vi "Get Diagnostics.vi"(8 "error in (no error)":errorcluster, 11 "Red Pitaya Digitizer in":refnum<class "Red Pitaya Digitizer.lvclass">) -> (0 "error out":errorcluster, 2 "Diagnostics":string, 3 "Red Pitaya Digitizer out":refnum<class "Red Pitaya Digitizer.lvclass">)   [LabVIEW 2024, in "Red Pitaya Digitizer.lvclass"]
uses:
  Red Pitaya Digitizer.lvclass
  RP Core/RP Instrument/RP Instrument.lvclass
  Red Pitaya Digitizer.lvclass/Red Pitaya Digitizer.ctl
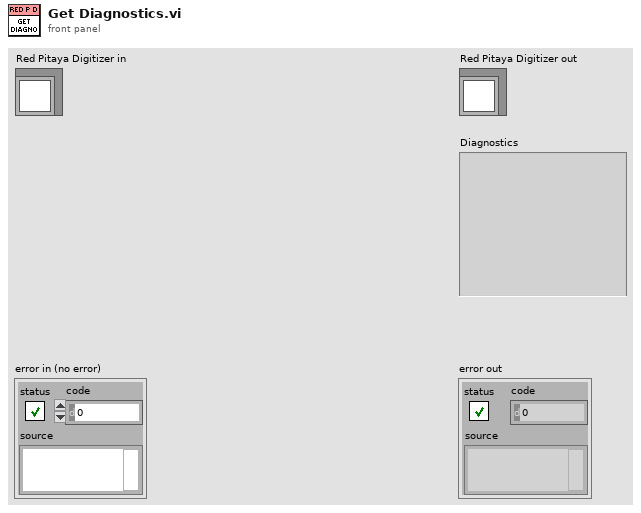
[diagram p1: front panel]
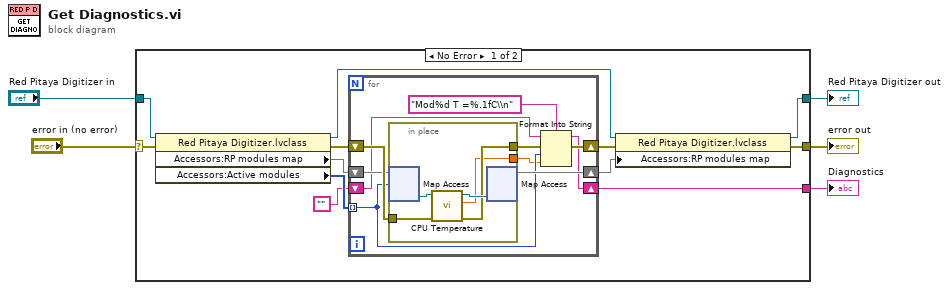
[diagram p0: block diagram]
diagram:
  n1 = case shown="No Error" "error in (no error)" {
    selector: "error in (no error)" -> [w14 w34]
    tunnel: "Red Pitaya Digitizer in" -> [w17 w33]
    tunnel: [w10 w33] -> w2
    tunnel: [w9 w34] -> w3
    tunnel: [w6 _] -> w1
    frame No Error {
      n2 = property class="Red Pitaya Digitizer.lvclass"(reference=w17, error in=w14) -> (reference out=w13:refnum<class "Red Pitaya Digitizer.lvclass">, error out=w15:errorcluster, "Accessors:RP modules map "=w16:map{i32, refnum<class "RP Instrument.lvclass">}, "Accessors:Active modules"=w8:i32[])
      n3 = for {
        shift-right: [w20] -> w12
        shift-left: w15 -> [w27]
        shift-right: [w25] -> w11
        shift-left: w16 -> [w26]
        tunnel: w8 -> [w23] mode=indexing
        shift-right: [w19] -> w6
        shift-left: "" -> [w18]
        n4 = in-place {
          in-place-border: w27 -> [w29]
          in-place-border: [w30] -> w21
          in-place-border: [w28] -> w22
          n5 = in-place-map #1(w26, w23) -> (w32:refnum<class "RP Instrument.lvclass">)  [unwired: 1 in, 1 out]
          n6 = call-dynamic "CPU Temperature.vi"("error in (no error)"=w29, "RP Instrument in"=w32) -> ("error out"=w30:errorcluster, "CPU Temperature"=w28:dbl, "RP Instrument out"=w31:refnum<class "RP Instrument.lvclass">)  [unwired: 7 in]
          n7 = in-place-map #1(w31) -> (w25:map{i32, refnum<class "RP Instrument.lvclass">})  [unwired: 1 in, 2 out]
        }
        n8 = Format Into String(format string="Mod%d T =%.1fC\\n", initial string=w18, error in=w21, w23, w22) -> (resulting string=w19:string, error out=w20:errorcluster)
      }
      n9 = property class="Red Pitaya Digitizer.lvclass"(reference=w13, error in=w12, "Accessors:RP modules map "=w11) -> (reference out=w10:refnum<class "Red Pitaya Digitizer.lvclass">, error out=w9:errorcluster)
    }
    frame Error {
    }
  }
  "error out" <- w3
  "Red Pitaya Digitizer out" <- w2
  "Diagnostics" <- w1
